vi "StringInputKeyboardSimulation.vi"(0 "VI Reference In":refnum<vi>, 5 "Control Path":string, 7 "string":string, 11 "Error In":errorcluster) -> (4 "VI Reference Out":refnum<vi>, 15 "Error Out":errorcluster)   [LabVIEW 2016, in "Drona.lvlib" / "KeyboardSimulation.lvlib"]
doc: "Convert the input string into key array and handle the actions configured for each of the keys in the control."
uses:
  KeyboardSimulation.lvlib
  typedef/VirtualKey.ctl
  typedef/Action.ctl
  user32.dll
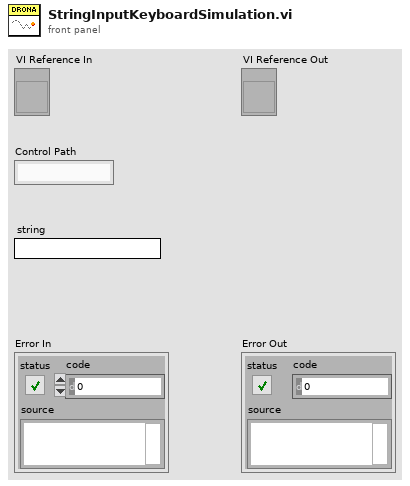
[diagram p1: front panel]
types:
  T1 = typedef "Drona.lvlib/KeyboardSimulation.lvlib/VirtualKey.ctl" = u8
  T2 = typedef "Drona.lvlib/KeyboardSimulation.lvlib/Action.ctl" = enum16{"Press", "Up", "Down"}
  T3 = cluster{"Key":T1, "Action":T2, "Delay (ms)":u32}[]
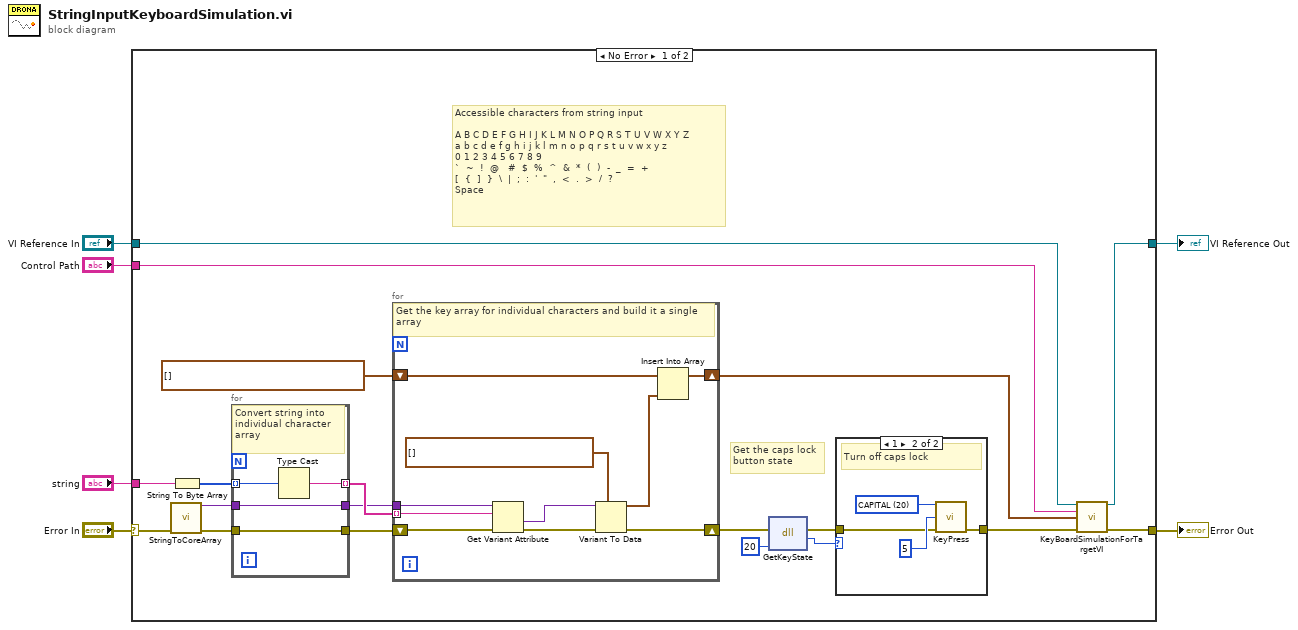
[diagram p0: block diagram]
diagram:
  n1 = case shown="No Error" "Error In" {
    selector: "Error In" -> [w22 w45]
    tunnel: "string" -> [w20 _]
    tunnel: "VI Reference In" -> [w15 w46]
    tunnel: "Control Path" -> [w14 _]
    tunnel: [w13 w46] -> w2
    tunnel: [w12 w45] -> w1
    frame No Error {
      # "Accessible characters from string input\n\nA B C D E F G H I J K L M N O P Q R S T U V W X Y Z \na b c d e f g h i j k l m n o p q r s t u v w x y z\n0 1 2 3 4 5 6 7 8 9\n`  ~  !  @   #  $  %  ^  &  *  (  )  -  _  =  + \n[  {  ]  }  \\  |  ;  :  '  \"  ,  <  .  >  /  ?\nSpace"
      # "Get the caps lock\nbutton state"
      n2 = call "StringToCoreArray.vi"("Error In"=w22) -> ("Key Value Variant"=w19:variant, "Error Out"=w21:errorcluster)  [unwired: 13 in]
      n3 = String To Byte Array(string=w20) -> (unsigned byte array=w25:u8[])
      n4 = for {
        tunnel: w25 -> [w44] mode=indexing
        tunnel: [w43] -> w24 mode=indexing
        tunnel: w21 -> [w42]
        tunnel: [w42] -> w17
        tunnel: w19 -> [w41]
        tunnel: [w41] -> w18
        # "Convert string into individual character array"
        n5 = Type Cast(x=w44) -> (*(type *) &x=w43:string)  [unwired: 1 in]
      }
      n6 = for {
        tunnel: w24 -> [w39] mode=indexing
        tunnel: w18 -> [w40]
        shift-right: [w34] -> w16
        shift-left: T3 [] ("Key Array") -> [w35]
        shift-right: [w37] -> w11
        shift-left: w17 -> [w31]
        # "Get the key array for individual characters and build it a single array"
        n7 = Get Variant Attribute(Variant=w40, name=w39, error in=w31) -> (value=w36:variant, error out=w38:errorcluster)  [unwired: 1 in, 2 out]
        n8 = Variant To Data(error in=w38, type=T3 [] ("Key Array"), Variant=w36) -> (data=w32:T3, error out=w37:errorcluster)
        n9 = Insert Into Array(array=w35, new element=w32) -> (w34:T3)  [unwired: 1 in]
      }
      n10 = dll-call lib="user32.dll" fn="GetKeyState"(error in=w11, "arg"=u8 20 ("Virtual Key")) -> (error out=w7:errorcluster, "return type"=w8:u8)  [unwired: 3 in, 1 out]
      n11 = case shown="1" w8 {
        tunnel: [w26 w30] -> w10
        tunnel: w7 -> [w26 w27]
        frame 0, Default {
          # "Caps lock is off"
        }
        frame 1 {
          w28 = T1 20 items=["LBUTTON"=1, "RBUTTON"=2, "CANCEL"=3, "MBUTTON"=4, "BACKSPACE"=8, "TAB"=9, "CLEAR"=12, "ENTER"=13, "SHIFT"=16, "CTRL"=17, "ALT"=18, "PAUSE"=19, "CAPITAL"=20, "ESCAPE"=27, "SPACE"=32, "PAGEUP"=33, "PAGEDOWN"=34, "END"=35, "HOME"=36, "LEFTARROW"=37, "UPARROW"=38, "RIGHTARROW"=39, "DOWNARROW"=40, "SELECT"=41, "PRINT"=42, "EXECUTE"=43, "PRINTSCREEN"=44, "INSERT"=45, "DELETE"=46, "HELP"=47, "0"=48, "1"=49, "2"=50, "3"=51, "4"=52, "5"=53, "6"=54, "7"=55, "8"=56, "9"=57, "A"=65, "B"=66, "C"=67, "D"=68, "E"=69, "F"=70, "G"=71, "H"=72, "I"=73, "J"=74, "K"=75, "L"=76, "M"=77, "N"=78, "O"=79, "P"=80, "Q"=81, "R"=82, "S"=83, "T"=84, "U"=85, "V"=86, "W"=87, "X"=88, "Y"=89, "Z"=90, "LWIN"=91, "RWIN"=92, "APPS"=93, "NUMPAD0"=96, "NUMPAD1"=97, "NUMPAD2"=98, "NUMPAD3"=99, "NUMPAD4"=100, "NUMPAD5"=101, "NUMPAD6"=102, "NUMPAD7"=103, "NUMPAD8"=104, "NUMPAD9"=105, "MULTIPLY"=106, "ADD"=107, "SEPERATOR"=108, "SUBTRACT"=109, "DECIMAL"=110, "DIVIDE"=111, "F1"=112, "F2"=113, "F3"=114, "F4"=115, "F5"=116, "F6"=117, "F7"=118, "F8"=119, "F9"=120, "F10"=121, "F11"=122, "F12"=123, "F13"=124, "F14"=125, "F15"=126, "F16"=127, "F17"=128, "F18"=129, "F19"=130, "F20"=131, "F21"=132, "F22"=133, "F23"=134, "F24"=135, "NUMLOCK"=144, "SCROLL"=145, "LSHIFT"=160, "RSHIFT"=161, "LCTRL"=162, "RCTRL"=163, "LALT"=164, "RALT"=165, "VOLMUTE"=173, "VOLDOWN"=174, "VOLUP"=175, ";    :"=186, "=   +"=187, ",    <"=188, "-    _"=189, ".    >"=190, "/    ?"=191, "`    ~"=192, "[    {"=219, "\\    |"=220, "]    }"=221, "'    \""=222] ("Virtual Key")
          # "Turn off caps lock"
          n12 = call "KeyPress.vi"("Virtual Key"=w28, "Millis"=u32 5, "error in"=w27) -> ("error out"=w30:errorcluster)  [unwired: 12 in]
        }
      }
      n13 = call "KeyBoardSimulationForTargetVI.vi"("VI Reference In"=w15, "Control Path"=w14, "Key Array"=w16, "error In"=w10) -> ("VI Reference Out"=w13:refnum<vi>, "error IO"=w12:errorcluster)  [unwired: 10 in]
    }
    frame Error {
    }
  }
  "VI Reference Out" <- w2
  "Error Out" <- w1
